vi "Actor Core.vi"(8 "error in":errorcluster, 11 "Base Software in":refnum<class "Main.lvclass">) -> (0 "error out":errorcluster, 3 "Actor out":refnum<class "Actor.lvclass">)   [LabVIEW 2023, in "Main.lvlib" / "Main.lvclass"]
doc: "The Main UI for JPL's Base Software"
uses:
  Project/Main.lvclass
  C:/Users/Public/Documents/Development/builds/Engine/Engine.lvlibp/Project/Engine.lvclass
  builds/Engine/Actor Framework.lvlibp/1abvi3w/vi.lib/ActorFramework/Actor/Actor.lvclass
  Base Software Messages/Respond to Menu Event Msg/Respond to Menu Event Msg.lvclass/Respond to Menu Event Msg.ctl
  Base Software Messages/Update System Status Msg/Update System Status Msg.lvclass/Update System Status Msg.ctl
  Base Software Messages/Process Test Name Event Msg/Process Test Name Event Msg.lvclass/Process Test Name Event Msg.ctl
  builds/Engine/Engine.lvlibp/Accessors/Write VI_Ref.vi
  Accessors/GUI/Write Splitters.vi
  builds/Engine/Actor Framework.lvlibp/1abvi3w/vi.lib/ActorFramework/Message Enqueuer/Enqueue.vi
  Base Software Messages/Respond to Menu Event Msg/Respond to Menu Event Msg.lvclass
  Base Software Messages/Update System Status Msg/Update System Status Msg.lvclass
  Base Software Messages/Process Test Name Event Msg/Process Test Name Event Msg.lvclass
  builds/Engine/Engine.lvlibp/Project/Engine.lvclass
panel:
  out "Powered Time":string="Enter UUT"
  out "Witness":string="Login"
  out "Operator":string="Login"
  out "Serial":string="Serial"
  out "Model":string="Model"
  out "Time Stamp":timestamp format="%<%X\n%x>T"
  out "Status":string
  in  "Stop":bool
  out "Version":string caption="v"
  in  "Open_Report":bool
  in  "UUT_Info":bool
  in  "Config":bool
  in  "Manual":bool
  in  "Login":bool
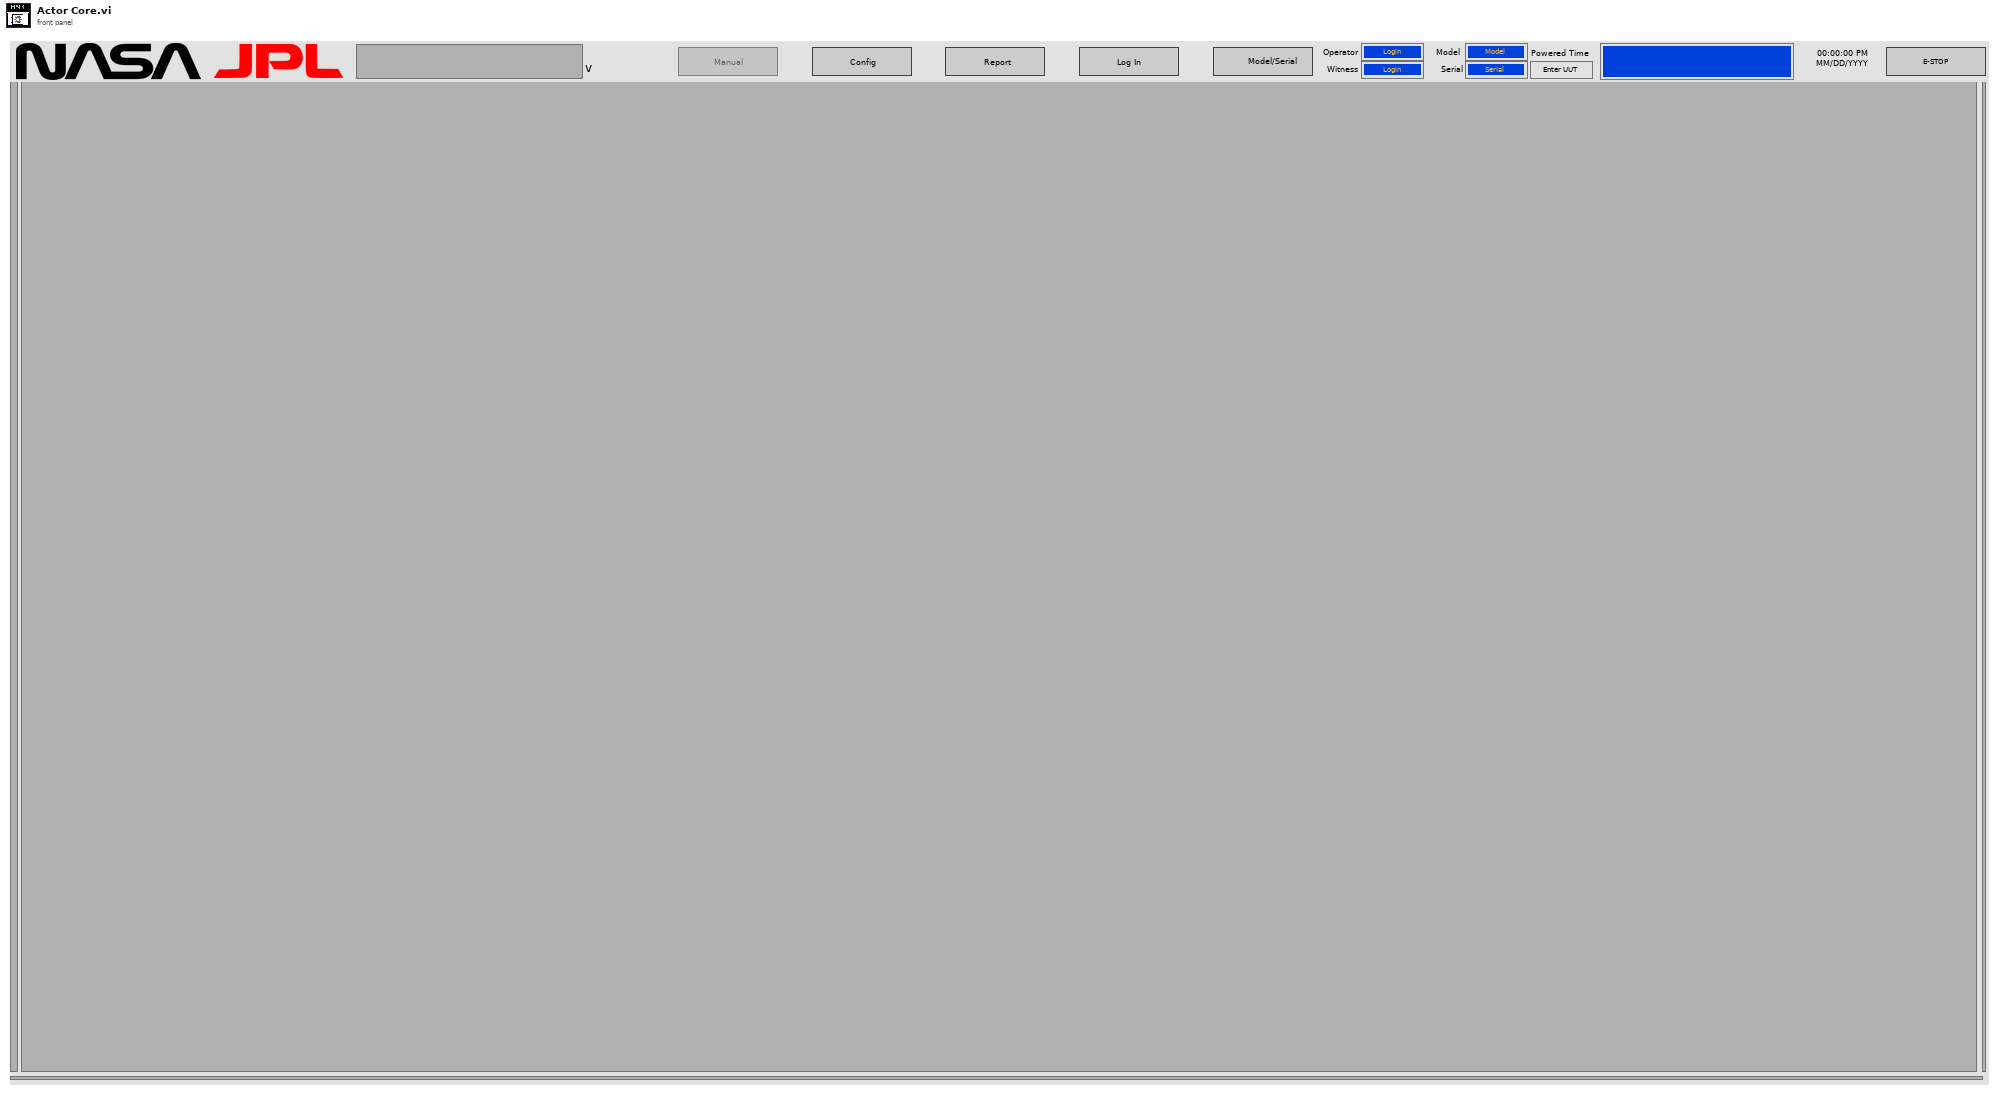
[diagram p1: front panel]
types:
  T1 = cluster{"Pnl Actor":refnum<event-registration>, "Event Registration Refnum":refnum<event-registration>}
  T2 = typedef "Engine.lvlibp/Engine.lvclass/System Status.ctl" = enum16{"Logged Off", "UUT_Info_Missing", "Idle", "Error", "Warning", "Loading", "Config", "Manual", "Automation", "Report_View", "Previous"}
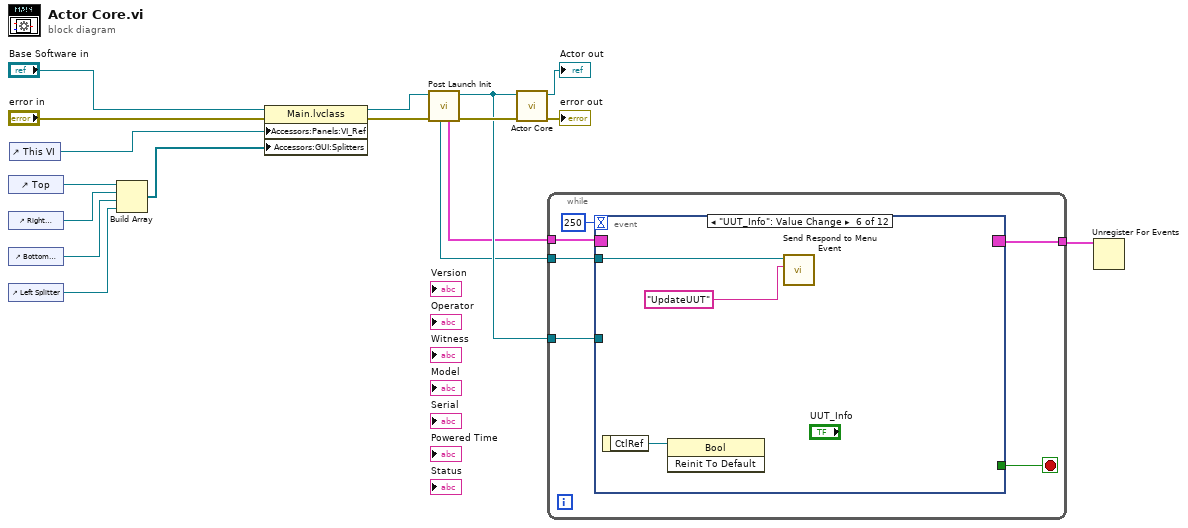
[diagram p0: block diagram]
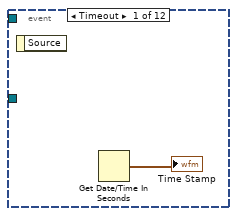
[diagram p2: hidden frame]
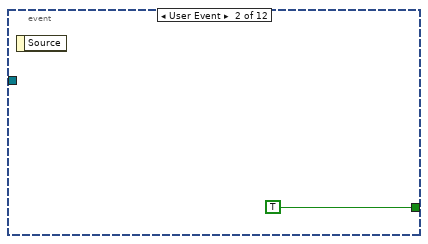
[diagram p3: hidden frame]
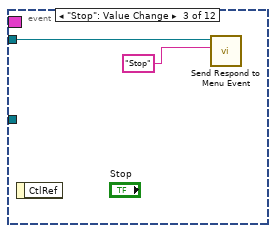
[diagram p4: hidden frame]
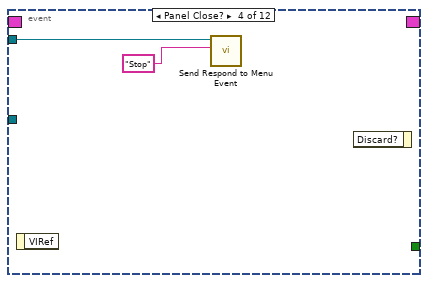
[diagram p5: hidden frame]
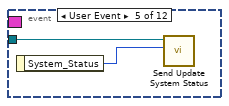
[diagram p6: hidden frame]
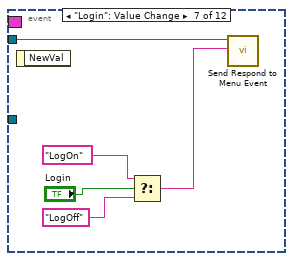
[diagram p7: hidden frame]
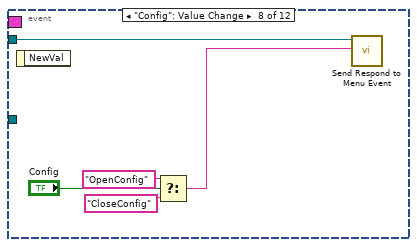
[diagram p8: hidden frame]
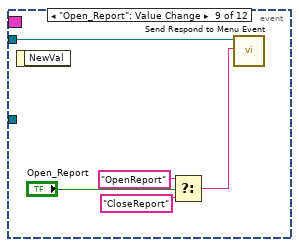
[diagram p9: hidden frame]
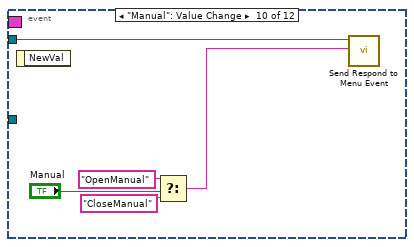
[diagram p10: hidden frame]
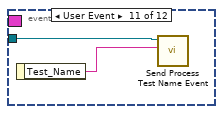
[diagram p11: hidden frame]
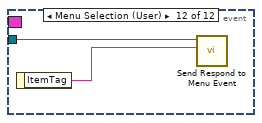
[diagram p12: hidden frame]
diagram:
  n1 = control-ref of="Top"() -> (w14:refnum<vi>)
  n2 = control-ref of="Right Splitter"() -> (w13:refnum<vi>)
  n3 = control-ref of="Bottom Splitter"() -> (w12:refnum<vi>)
  n4 = control-ref of="Left Splitter"() -> (w11:refnum<vi>)
  n5 = control-ref of="This VI"() -> (w1:refnum<vi>)
  n6 = Build Array(w14, w13, w12, w11) -> (w10:refnum<vi>[])
  n7 = property class="Main.lvclass"(reference="Base Software in", error in="error in", "Accessors:Panels:VI_Ref"=w1, "Accessors:GUI:Splitters"=w10) -> (reference out=w6:refnum<class "Main.lvclass">, error out=w7:errorcluster)
  n8 = call "Post Launch Init.vi"("error in"=w7, "Base Software in"=w6) -> ("error out"=w8:errorcluster, "Base Software out"=w5:refnum<class "Main.lvclass">, "Events"=w4:T1, "Self Enqueuer"=w2:refnum<class "Message Enqueuer.lvclass">)  [unwired: 6 in]
  n9 = call-parent "Actor Core.vi"("error in"=w8, "State Actor in"=w5) -> ("error out"=→"error out":errorcluster, "Actor out"=→"Actor out":refnum<class "Actor.lvclass">)  [unwired: 8 in]
  n10 = while {
    tunnel: w2 -> [w22]
    tunnel: w5 -> [w21]
    tunnel: w4 -> [w20]
    tunnel: [w19] -> w3
    stop <- w23 stop-if-true
    n11 = event shown="[5] \"UUT_Info\": Value Change" {
      selector: w20 -> [_ _ _ _ _ _ _ _ _ _ _ _]
      dyn-events: [_ _ _ _ _ _ _ _ _ _ _ _] -> w19
      timeout: 250 -> [_ _ _ _ _ _ _ _ _ _ _ _]
      tunnel: [_ TRUE _ _ _ _ _ _ _ _ _ _] -> w23
      tunnel: w22 -> [_ _ w27 w29 w31 w33 w36 w41 w46 w51 w56 w58]
      tunnel: w21 -> [_ _ _ _ _ _ _ _ _ _ _ _]
      event Timeout {
        n12 = event-data() -> ()  [unwired: 1 in, 1 out]
        n13 = Get Date/Time In Seconds() -> (seconds since 1Jan1904=→"Time Stamp":timestamp)
      }
      event User Event {
        n14 = event-data() -> ()  [unwired: 1 in, 1 out]
      }
      event "Stop": Value Change {
        n15 = event-data() -> ()  [unwired: 1 in, 1 out]
        n16 = call "Send Respond to Menu Event.vi"("Selection"="Stop", "Message Enqueuer"=w27) -> ()  [unwired: 8 in, 2 out]
      }
      event Panel Close? {
        n17 = event-data() -> ()  [unwired: 1 in, 1 out]
        n18 = call "Send Respond to Menu Event.vi"("Selection"="Stop", "Message Enqueuer"=w29) -> ()  [unwired: 8 in, 2 out]
        n19 = event-data() -> ()  [unwired: 2 in, 1 out]
      }
      event User Event {
        n20 = event-data() -> ("System_Status"=w30:T2)  [unwired: 1 in]
        n21 = call "Send Update System Status.vi"("System_Status"=w30, "Message Enqueuer"=w31) -> ()  [unwired: 8 in, 2 out]
      }
      event "UUT_Info": Value Change {
        n22 = event-data() -> ("CtlRef"=w34:refnum<vi>)  [unwired: 1 in]
        n23 = invoke class="Bool" method="Reinit To Default"(reference=w34) -> ()  [unwired: 2 in, 3 out]
        n24 = call "Send Respond to Menu Event.vi"("Selection"="UpdateUUT", "Message Enqueuer"=w33) -> ()  [unwired: 8 in, 2 out]
      }
      event "Login": Value Change {
        n25 = event-data() -> ()  [unwired: 1 in, 1 out]
        n26 = Select(t="LogOn" ("Selection"), s="Login", f="LogOff" ("Selection")) -> (s? t:f=w35:string)
        n27 = call "Send Respond to Menu Event.vi"("Selection"=w35, "Message Enqueuer"=w36) -> ()  [unwired: 8 in, 2 out]
      }
      event "Config": Value Change {
        n28 = event-data() -> ()  [unwired: 1 in, 1 out]
        n29 = Select(t="OpenConfig", s="Config", f="CloseConfig" ("t")) -> (s? t:f=w40:string)
        n30 = call "Send Respond to Menu Event.vi"("Selection"=w40, "Message Enqueuer"=w41) -> ()  [unwired: 8 in, 2 out]
      }
      event "Open_Report": Value Change {
        n31 = event-data() -> ()  [unwired: 1 in, 1 out]
        n32 = Select(t="OpenReport", s="Open_Report", f="CloseReport" ("t")) -> (s? t:f=w45:string)
        n33 = call "Send Respond to Menu Event.vi"("Selection"=w45, "Message Enqueuer"=w46) -> ()  [unwired: 8 in, 2 out]
      }
      event "Manual": Value Change {
        n34 = event-data() -> ()  [unwired: 1 in, 1 out]
        n35 = Select(t="OpenManual", s="Manual", f="CloseManual" ("t")) -> (s? t:f=w50:string)
        n36 = call "Send Respond to Menu Event.vi"("Selection"=w50, "Message Enqueuer"=w51) -> ()  [unwired: 8 in, 2 out]
      }
      event User Event {
        n37 = event-data() -> ("Test_Name"=w55:string)  [unwired: 1 in]
        n38 = call "Send Process Test Name Event.vi"("TestName"=w55, "Message Enqueuer"=w56) -> ()  [unwired: 8 in, 2 out]
      }
      event Menu Selection (User) {
        n39 = event-data() -> ("ItemTag"=w57:string)  [unwired: 1 in]
        n40 = call "Send Respond to Menu Event.vi"("Selection"=w57, "Message Enqueuer"=w58) -> ()  [unwired: 8 in, 2 out]
      }
    }
  }
  n41 = Unregister For Events(event registration refnum=w3) -> ()  [unwired: 1 in, 1 out]
